vi "Launch Results UI.vi"(8 "error in (no error)":errorcluster, 10 "uniqueresultsid":string, 11 "Controller in":refnum<class "Controller.lvclass">) -> (0 "error out":errorcluster, 3 "Controller out":refnum<class "Controller.lvclass">)   [LabVIEW 2017, in "Controller Actor.lvlib" / "Controller.lvclass"]
uses:
  Controller.lvclass
  C:/Program Files (x86)/National Instruments/LabVIEW 2017/vi.lib/ActorFramework/Actor/Actor.lvclass
  Results/Results.lvclass
  <vilib>/ActorFramework/Actor/Actor.lvclass/Actor.ctl
  <vilib>/ActorFramework/Message Enqueuer/Message Enqueuer.lvclass/Message Enqueuer.ctl
  <vilib>/ActorFramework/Message Enqueuer/Init from Existing Queue.vi
  <vilib>/ActorFramework/Message Enqueuer/Enqueue.vi
  <vilib>/ActorFramework/Stop Msg/Stop Msg.lvclass
  C:/Program Files (x86)/National Instruments/LabVIEW 2017/vi.lib/ActorFramework/Message/Message.lvclass
  <vilib>/ActorFramework/Message Priority Queue/Priority Enqueue.vi
  <vilib>/ActorFramework/Message Enqueuer/Message Enqueuer.lvclass
  <vilib>/ActorFramework/Actor/Actor.lvclass
  Results/Messages/Display Results Msg/Display Results Msg.lvclass
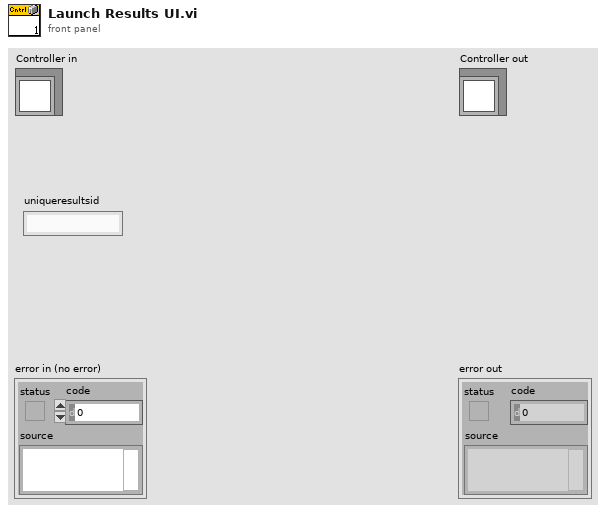
[diagram p1: front panel]
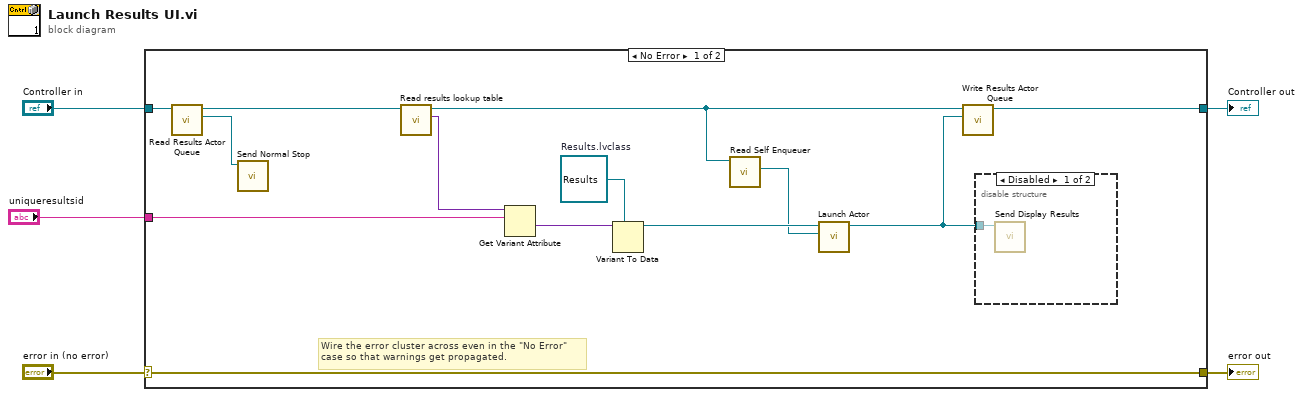
[diagram p0: block diagram]
diagram:
  n1 = case shown="No Error" "error in (no error)" {
    selector: "error in (no error)" -> [w18 w21]
    tunnel: [w18 w21] -> w4
    tunnel: [w10 w20] -> w2
    tunnel: "Controller in" -> [w12 w20]
    tunnel: "uniqueresultsid" -> [w16 _]
    frame No Error {
      w14 = refnum<class "Results.lvclass"> refnum  # Results.lvclass
      # "Wire the error cluster across even in the \"No Error\"\ncase so that warnings get propagated."
      n2 = call "Read Results Actor Queue.vi"("Controller in"=w12) -> ("Message Enqueuer"=w8:refnum<class "Message Enqueuer.lvclass">, "Controller out"=w11:refnum<class "Controller.lvclass">)  [unwired: 8 in, 1 out]
      n3 = call <vilib>:"Send Normal Stop.vi"("Message Enqueuer"=w8) -> ()  [unwired: 10 in, 1 out]
      n4 = call "Read results lookup table.vi"("Controller in"=w11) -> ("results lookup table (measurement.timestamp -> results object)"=w17:variant, "Controller out"=w7:refnum<class "Controller.lvclass">)  [unwired: 8 in, 1 out]
      n5 = Get Variant Attribute(Variant=w17, name=w16) -> (value=w15:variant)  [unwired: 2 in, 3 out]
      n6 = Variant To Data(type=w14, Variant=w15) -> (data=w13:refnum<class "Results.lvclass">)  [unwired: 1 in, 1 out]
      n7 = call <vilib>:"Read Self Enqueuer.vi"("Actor"=w7) -> ("Self Enqueuer"=w6:refnum<class "Message Enqueuer.lvclass">)  [unwired: 10 in]
      n8 = call <vilib>:"Launch Actor.vi"("Actor-to-Caller Enqueuer"=w6, "Actor"=w13) -> ("Caller-To-Actor Enqueuer"=w9:refnum<class "Message Enqueuer.lvclass">)  [unwired: 8 in, 1 out]
      n9 = call "Write Results Actor Queue.vi"("Message Enqueuer in"=w9, "Controller in"=w7) -> ("Controller out"=w10:refnum<class "Controller.lvclass">)  [unwired: 8 in, 1 out]
      n10 = disable-structure shown="Disabled" {
        disable-tunnel: w9 -> [w19 _]
        frame Disabled {
          n11 = call "Send Display Results.vi"("Message Enqueuer in"=w19) -> ()  [unwired: 9 in, 2 out]
        }
        frame Enabled {
        }
      }
    }
    frame Error {
    }
  }
  "error out" <- w4
  "Controller out" <- w2
